vi "GetDescendants.vi"(8 "error in":errorcluster, 11 "node in":refnum<data-value>) -> (0 "error out":errorcluster, 3 "descendants":refnum<data-value>[](array[refnum]))   [LabVIEW 2013, in "NISE_CEF_Node.lvclass"]
uses:
  NISE_CEF_Node.lvclass
  NISE_CEF_Node.lvclass/NISE_CEF_Node.ctl
  ReadChildren.vi
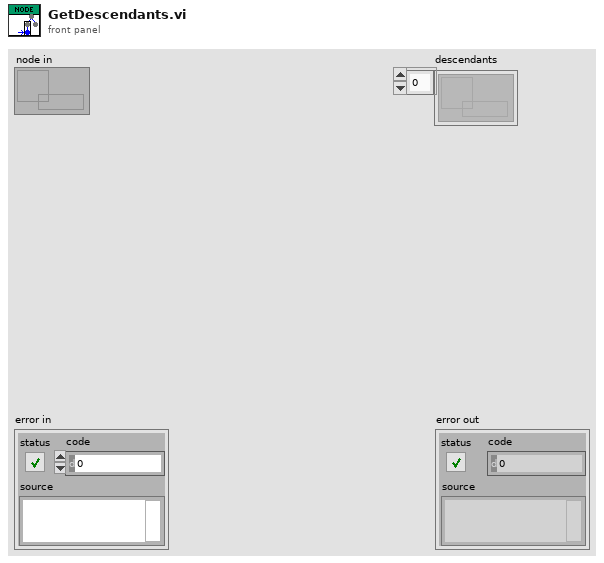
[diagram p1: front panel]
types:
  T1 = typedef "NISE_CEF_Node.lvclass/NodeRef.ctl" = refnum<data-value>
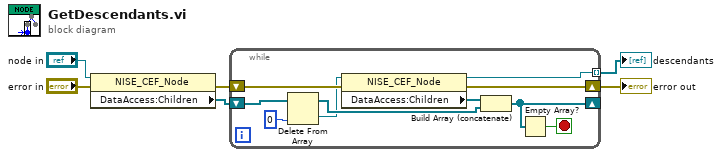
[diagram p0: block diagram]
diagram:
  n1 = property class="NISE_CEF_Node"(reference="node in", error in="error in") -> (error out=w3:errorcluster, "DataAccess:Children"=w4:T1[])  [unwired: 1 out]
  n2 = while {
    shift-right: [w9] -> _
    shift-left: w4 -> [w16]
    shift-right: [w13] -> w2
    shift-left: w3 -> [w14]
    tunnel: [w7] -> w1 mode=indexing
    stop <- w8 stop-if-true
    n3 = Delete From Array(array=w16, index=0) -> (deleted portion=w11:T1, array with subset deleted=w12:T1[])  [unwired: 1 in]
    n4 = property class="NISE_CEF_Node"(reference=w11, error in=w14) -> (reference out=w7:T1, error out=w13:errorcluster, "DataAccess:Children"=w10:T1[])
    n5 = Build Array (concatenate)(w10, w12) -> (w9:T1[])
    n6 = Empty Array?(array=w9) -> (empty?=w8:bool)
  }
  "error out" <- w2
  "descendants" <- w1
